vi "editscenario.vi"(7 "httpRequestID":u32) -> ()   [LabVIEW 2011]
doc: "This VI is a state machine that can be ran from a Browser."
uses:
  server/database/Users/User Record.ctl
  <vilib>/addons/internet/utils/strutil.llb/Case Matching.ctl
  <vilib>/wsapi/NI_WebServices.lvlib
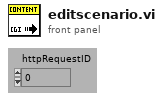
[diagram p1: front panel]
types:
  T1 = typedef "User Record.ctl" = cluster{"ixUser":i32, "sxUsername":string, "sLastName":string, "sFirstName":string, "sEmail":string, "sPassword":string, "tLoginTime":timestamp, "sLoginComputer":string, "fAdministrator":bool, "fRunSequences":bool, "fModifySequences":bool, "fRunScenarios":bool, "fModifyScenarios":bool, "fModifyTemplates":bool, "fModifyUsers":bool, "fModifyStations":bool, "fModifyFields":bool}
  T2 = typedef "Connection Refnum.ctl" = cluster{"Environment Handle":i32, "Connection Handle":i32}
  T3 = typedef "Case Matching.ctl" = enum16{"a != A", "a == A", "system"}
  T4 = typedef "Keyed Array.ctl" = cluster{"keys":string[], "values":string[]}
  T5 = cluster{"Local File Path":string, "Client File Name":string, "Content Type":string, "Size":u32}[]
  T6 = typedef "Scenario Record.ctl" = cluster{"ixScenario":i32, "tCreated":timestamp, "tModified":timestamp, "sxUsername":string, "sModifiedBy":string, "sxScenarioId":string, "sDescription":string, "sLogic":string, "sResultFieldsCSV":string, "sTemplatesCSV":string, "fAutoRunReports":bool, "fSortByTemplates":bool, "fCombinePDF":bool, "Conditions":T7[]}
  T7 = typedef "Condition Record.ctl" = cluster{"iConditionIndex":i32, "sxFieldId":string, "nOperator":T8, "sMatchValue":string}
  T8 = typedef "Condition Operators.ctl" = enum16{"equal (=)", "not equal (\\u2260)", "less than (<)", "less than or equal (\\u2264)", "greater than (>)", "greater than or equal (\\u2265)", "contains", "does not contain"}
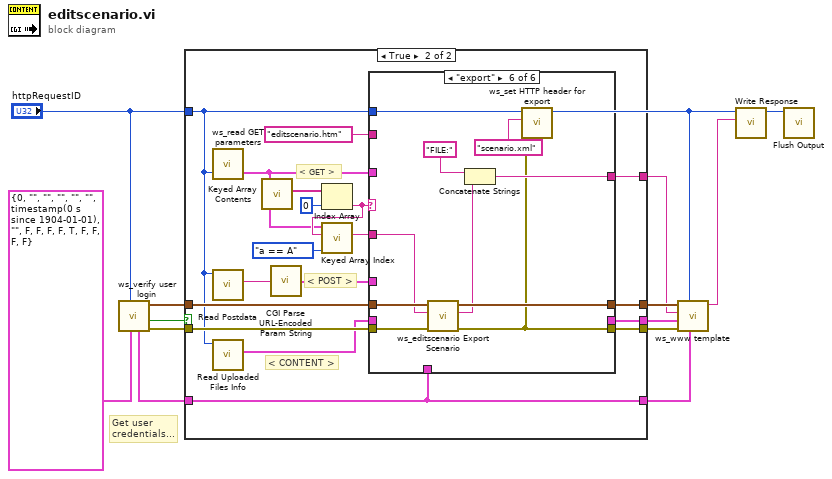
[diagram p0: block diagram]
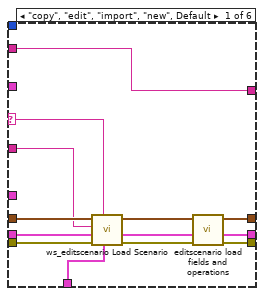
[diagram p3: hidden frame]
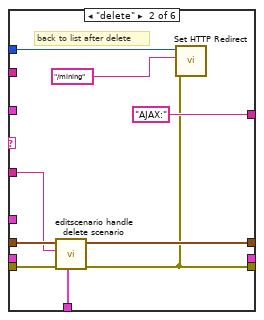
[diagram p4: hidden frame]
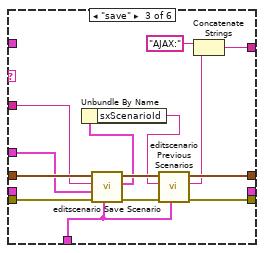
[diagram p5: hidden frame]
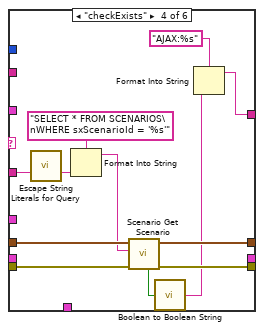
[diagram p6: hidden frame]
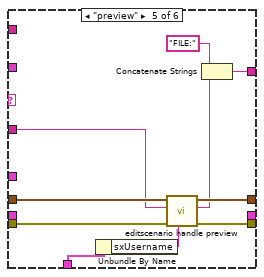
[diagram p7: hidden frame]
diagram:
  # "Get user \ncredentials..."
  n1 = call "ws_verify user login.vi"("Required Permisions"=T1 {"ixUser"=0, "sxUsername"="", "sLastName"="", "sFirstName"="", "sEmail"="", "sPassword"="", "tLoginTime"=timestamp(0 s since 1904-01-01), "sLoginComputer"="", "fAdministrator"=FALSE, "fRunSequences"=FALSE, "fModifySequences"=FALSE, "fRunScenarios"=FALSE, "fModifyScenarios"=TRUE, "fModifyTemplates"=FALSE, "fModifyUsers"=FALSE, "fModifyStations"=FALSE, "fModifyFields"=FALSE} ("User Record"), "httpRequestID"="httpRequestID") -> ("error out"=w13:errorcluster, "User Verified\nand Spartan\nAuthorized?"=w9:bool, "DB Connection Ref"=w10:T2, "User"=w11:T1)  [unwired: 6 in]
  n2 = case shown="True" w9 {
    tunnel: [w16 w23] -> w8
    tunnel: w13 -> [w16 w25]
    tunnel: w10 -> [w14 w26]
    tunnel: w11 -> [w15 w27]
    tunnel: [w15 w27] -> w5
    tunnel: [w14 w21] -> w7
    tunnel: [_ w20] -> w4
    tunnel: [_ w22] -> w6
    tunnel: "httpRequestID" -> [_ w17]
    frame False {
    }
    frame True {
      # "< CONTENT >"
      # "< GET >"
      # "< POST >"
      n3 = call "ws_read GET parameters.vi"("httpRequestID"=w17) -> ("GET query params"=w24:T4)  [unwired: 2 in]
      n4 = call <vilib>:"Read Postdata.vi"("httpRequestID"=w17) -> ("postdata"=w19:string)  [unwired: 8 in, 2 out]
      n5 = call <vilib>:"Read Uploaded Files Info.vi"("httpRequestID"=w17) -> ("UploadedFilesList"=w18:T5)  [unwired: 8 in, 2 out]
      n6 = call <vilib>:"Keyed Array Contents.vi"("array in"=w24) -> ("keys"=w34:string[])  [unwired: 4 in, 2 out]
      n7 = call <vilib>:"CGI Parse URL-Encoded Param String.vi"("url-encoded param string"=w19) -> ("params"=w32:T4)
      n8 = Index Array(array=w34, index=0) -> (element=w29:string)
      n9 = call <vilib>:"Keyed Array Index.vi"("case matching (sensitive)"=Case_Matching."a == A", "key"=w29, "array in"=w24) -> ("value"=w28:string)  [unwired: 1 in, 3 out]
      n10 = case shown="\"export\"" w29 {
        selector: w29 -> [w36 _ _ _ _ _]
        tunnel: w25 -> [w41 w54 w70 w81 w90 w98]
        tunnel: [w45 w48 w63 w76 w86 w93] -> w23
        tunnel: [w44 _ _ _ _ _] -> w22
        tunnel: [w46 w51 w64 w77 w88 w99] -> w21
        tunnel: w26 -> [w42 w55 w69 w82 w89 w100]
        tunnel: w27 -> [w43 w52 w61 _ w84 _]
        tunnel: w24 -> [_ _ _ _ _ _]
        tunnel: [w47 "AJAX:" ("Template (\"\")") w66 w73 w91 w101] -> w20
        tunnel: w32 -> [_ _ w68 _ _ _]
        tunnel: "editscenario.htm" ("Template (\"\")") -> [w47 _ _ _ _ _]
        tunnel: w28 -> [w37 w53 w60 w78 w87 w97]
        tunnel: w18 -> [w35 _ _ _ _ _]
        tunnel: w17 -> [_ w50 _ _ _ w94]
        frame "copy", "edit", "import", "new", Default {
          n11 = call "ws_editscenario Load Scenario.vi"("User Information"=w43, "command (\"edit\")"=w36, "error in (no error)"=w41, "UploadedFilesList"=w35, "sxScenarioId (\"\")"=w37, "Connection Refnum"=w42) -> ("error out"=w40:errorcluster, "Template Keys"=w38:T4, "Connection Refnum"=w39:T2)  [unwired: 1 in, 2 out]
          n12 = call "editscenario load fields and operations.vi"("error in (no error)"=w40, "Template Keys (empty)"=w38, "Connection Refnum"=w39) -> ("error out"=w45:errorcluster, "Template Keys"=w44:T4, "Connection Refnum"=w46:T2)  [unwired: 6 out]
        }
        frame "delete" {
          # "back to list after delete"
          n13 = call "editscenario handle delete scenario.vi"("User Information"=w52, "error in (no error)"=w54, "scenarioId (\"\")"=w53, "Connection Refnum"=w55) -> ("error out"=w48:errorcluster, "Connection Refnum"=w51:T2)  [unwired: 6 out]
          n14 = call <vilib>:"Set HTTP Redirect.vi"("error in (no error)"=w48, "redirect URL"="/mining" ("New URL (testing.vit)"), "httpRequestID"=w50) -> ()  [unwired: 7 in, 2 out]
        }
        frame "save" {
          n15 = call "editscenario Save Scenario.vi"("User Information"=w61, "error in (no error)"=w70, "Save POST"=w68, "scenarioId (\"\")"=w60, "Connection Refnum"=w69) -> ("error out"=w62:errorcluster, "New Scenario"=w58:T6, "Connection Refnum"=w65:T2)  [unwired: 4 out]
          n16 = Unbundle By Name(w58) -> ("sxScenarioId"=w57:string)
          n17 = call "editscenario Previous Scenarios.vi"("User Information"=w61, "error in (no error)"=w62, "sxScenarioId (\"\")"=w57, "Connection Refnum"=w65) -> ("error out"=w63:errorcluster, "Previous SCENARIOS array"=w59:string, "Connection Refnum"=w64:T2)  [unwired: 5 out]
          n18 = Concatenate Strings("AJAX:" ("Template (\"\")"), w59) -> (w66:string)
        }
        frame "checkExists" {
          n19 = call "Escape String Literals for Query.vi"("String"=w78) -> ("escaped String"=w79:string)  [unwired: 1 in, 13 out]
          n20 = Format Into String(format string="SELECT * FROM SCENARIOS\nWHERE sxScenarioId = '%s'", w79) -> (resulting string=w75:string)  [unwired: 2 in, 1 out]
          n21 = call "Scenario Get Scenario.vi"("error in (no error)"=w81, "Query"=w75, "Connection Refnum"=w82) -> ("error out"=w76:errorcluster, "Connection Refnum"=w77:T2, "Data Present?"=w72:bool)  [unwired: 6 out]
          n22 = call "Boolean to Boolean String.vi"("Boolean"=w72) -> ("Boolean string"=w71:string)  [unwired: 1 in]
          n23 = Format Into String(format string="AJAX:%s" ("Template (\"\")"), w71) -> (resulting string=w73:string)  [unwired: 2 in, 1 out]
        }
        frame "preview" {
          n24 = Unbundle By Name(w84) -> ("sxUsername"=w83:string)
          n25 = call "editscenario handle preview.vi"("user"=w83, "error in (no error)"=w90, "sxScenarioId (\"\")"=w87, "Connection Refnum"=w89) -> ("error out"=w86:errorcluster, "image"=w85:string, "dup Connection Refnum"=w88:T2)  [unwired: 5 out]
          n26 = Concatenate Strings("FILE:" ("Template (\"\")"), w85) -> (w91:string)
        }
        frame "export" {
          n27 = call "ws_editscenario Export Scenario.vi"("error in (no error)"=w98, "sxScenarioId (\"\")"=w97, "Connection Refnum"=w100) -> ("error out"=w93:errorcluster, "scenario XML"=w96:string, "Connection Refnum"=w99:T2)  [unwired: 6 in]
          n28 = Concatenate Strings("FILE:" ("Template (\"\")"), w96) -> (w101:string)
          n29 = call "ws_set HTTP header for export.vi"("error in (no error)"=w93, "filename (\"\")"="scenario.xml" ("Template (\"\")"), "httpRequestID"=w94) -> ()  [unwired: 1 in, 8 out]
        }
      }
    }
  }
  n30 = call "ws_www template.vi"("User"=w5, "httpRequestID"="httpRequestID", "error in (no error)"=w8, "Template Keys (empty)"=w6, "Template (\"\")"=w4, "DB Connection Ref"=w7) -> ("HTTP Template Content"=w3:string)  [unwired: 5 in]
  n31 = call <vilib>:"Write Response.vi"("response string"=w3, "httpRequestID"="httpRequestID") -> ("httpRequestID out"=w1:u32)  [unwired: 8 in, 1 out]
  n32 = call <vilib>:"Flush Output.vi"("httpRequestID"=w1) -> ()  [unwired: 9 in, 2 out]
